vi "Vision Acquistion test.vi"() -> ()   [LabVIEW 2018]
uses:
  <vilib>/vision/driver/NI_Vision_Acquisition_Software.lvlib
panel:
  out "error out":errorcluster
  in  "error in":errorcluster
  in  "Stop (F)":bool
  out "Image Out":T1(plugin-control)
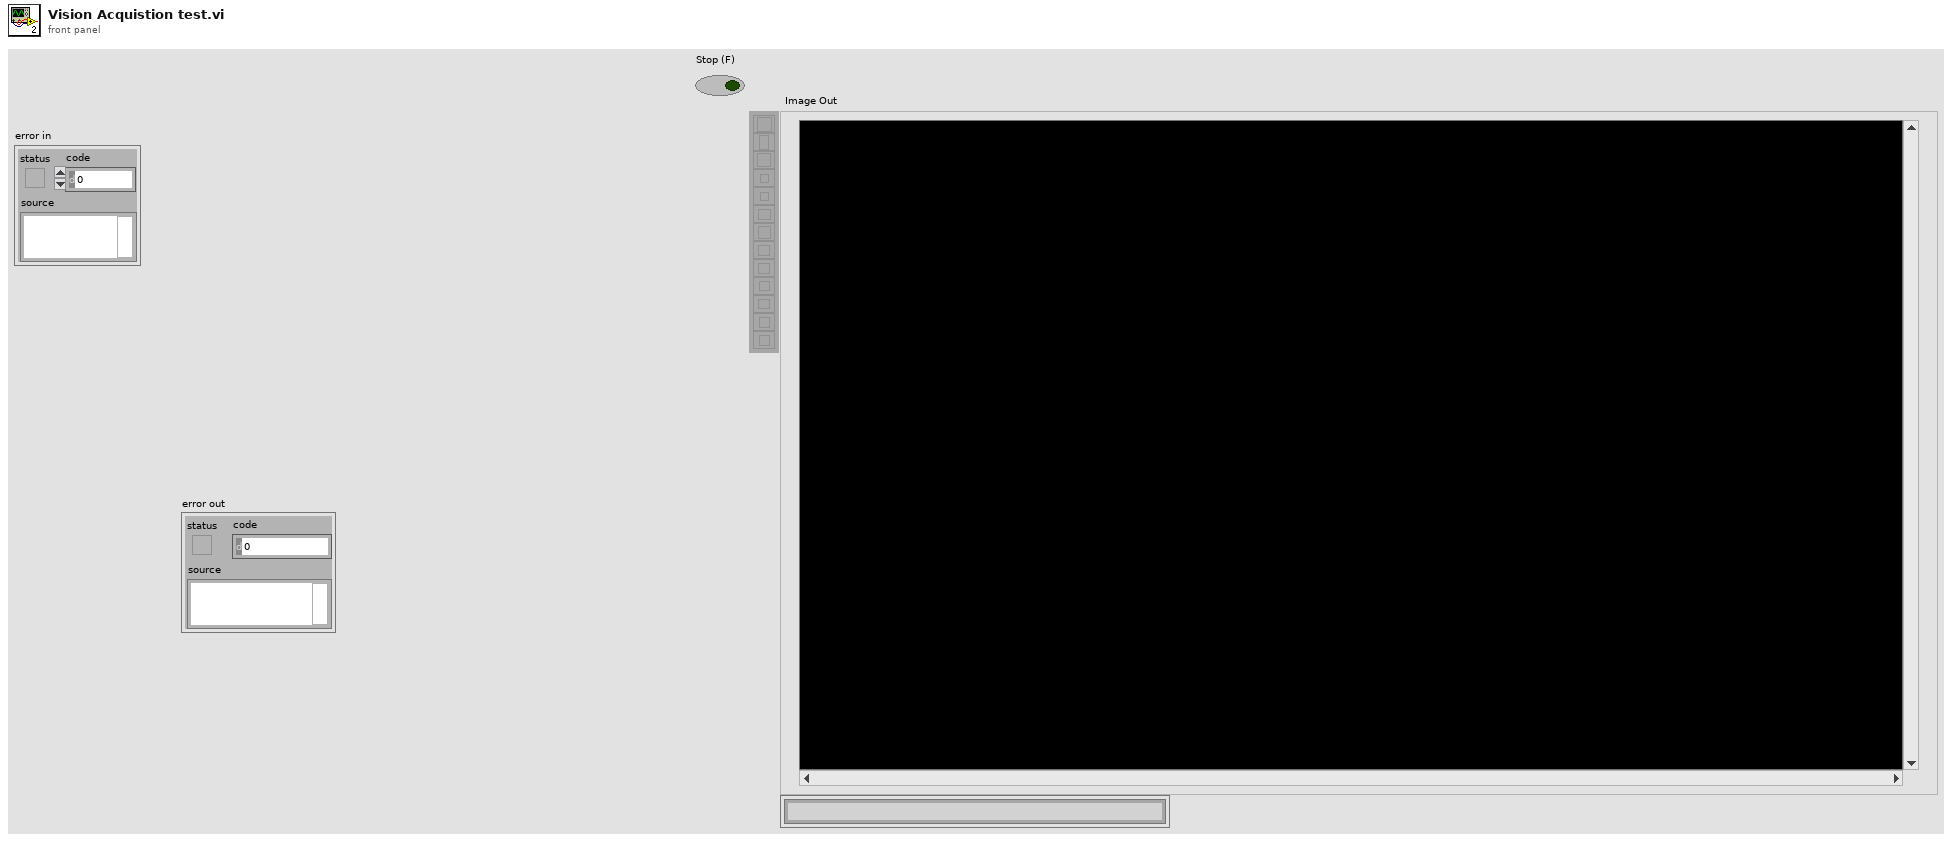
[diagram p1: front panel]
types:
  T1 = typedef "IMAQ Image.ctl" = refnum<image>
  T2 = typedef "IMAQdx.ctl" = refnum<k21>
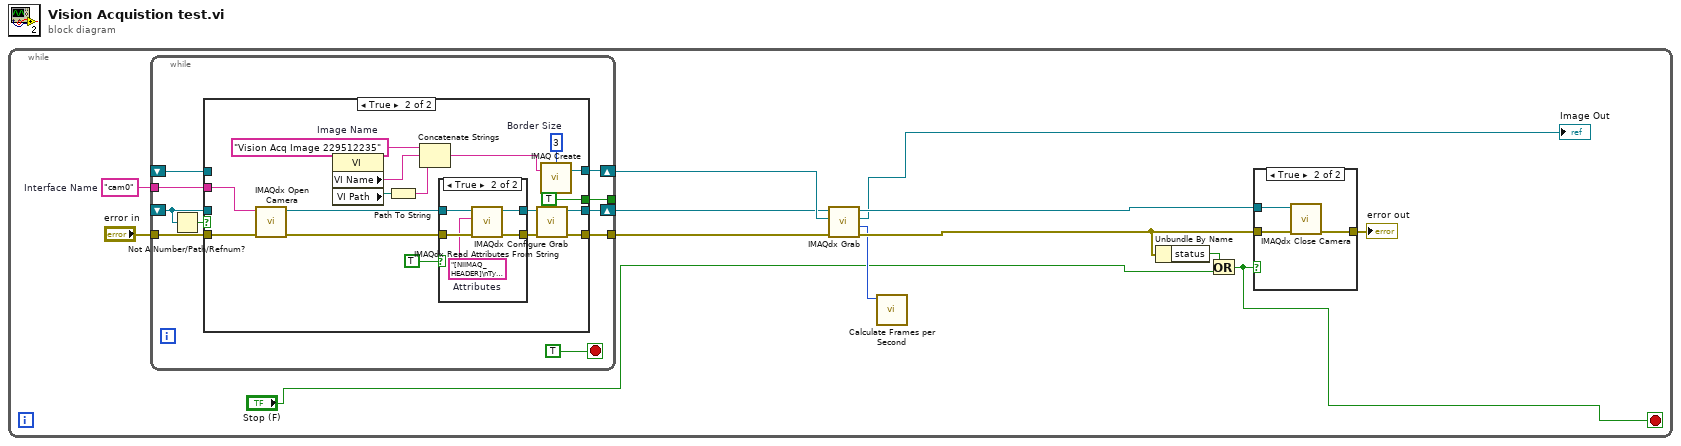
[diagram p0: block diagram]
diagram:
  n1 = while {
    stop <- w2 stop-if-true
    w11 = "cam0"  # Interface Name
    n2 = while "While Loop_template0" {
      shift-right: [w27] -> w9
      shift-left: _ -> [w20]
      tunnel: [w26] -> w12
      tunnel: "error in" -> [w25]
      shift-right: [w23] -> w10
      shift-left: _ -> [w22]
      tunnel: w11 -> [w21]
      tunnel: [w18] -> _
      stop <- TRUE ("_template0") stop-if-true
      n3 = Not A Number/Path/Refnum?(number/path/refnum=w20) -> (NaN/Path/Refnum?=w19:bool)
      n4 = case "Case Structure_template0" shown="True" w19 {
        tunnel: [w30 w46] -> w27
        tunnel: w20 -> [w30 _]
        tunnel: [w29 w45] -> w26
        tunnel: w25 -> [w29 w47]
        tunnel: [w28 w44] -> w23
        tunnel: w22 -> [w28 _]
        tunnel: w21 -> [_ w34]
        tunnel: [_ TRUE] -> w18
        frame False {
        }
        frame True {
          w31 = 3  # Border Size
          w39 = "Vision Acq Image 229512235"  # Image Name
          n5 = call <vilib>:"IMAQdx Open Camera.vi"("error in"=w47, "Session In"=w34) -> ("error out"=w37:errorcluster, "Session Out"=w38:T2)  [unwired: 1 in, 7 out]
          n6 = property class="VI"() -> ("VI Name"=w42:string, "VI Path"=w43:path)  [unwired: 2 in, 2 out]
          n7 = Path To String(path=w43) -> (string=w41:string)
          n8 = Concatenate Strings(w39, w42, w41) -> (w40:string)
          n9 = case shown="True" TRUE ("Init Attributes") {
            tunnel: w38 -> [w49 w54]
            tunnel: w37 -> [w48 w53]
            tunnel: [w49 w51] -> w36
            tunnel: [w48 w50] -> w35
            frame False {
            }
            frame True {
              w52 = "[NIIMAQ_HEADER]\nType = 2\nVersion = 8\n\n[CAMERA_DATA]\nAcquisitionAttributes::Bayer::Algorithm = \"Bilinear\"\nAcquisitionAttributes::Bayer::GainB = \"1\"\nAcquisitionAttributes::Bayer::GainG = \"1\"\nAcquisitionAttributes::Bayer::GainR = \"1\"\nAcquisitionAttributes::Bayer::Pattern = \"Use hardware value\"\nAcquisitionAttributes::BitsPerPixel = \"Use hardware value\"\nAcquisitionAttributes::HardwareMaximumQueuedBufferCount = \"1000\"\nAcquisitionAttributes::HardwareRequeueBufferListThreshold = \"50\"\nAcquisitionAttributes::IgnoreFirstFrame = \"false\"\nAcquisitionAttributes::ImageDecoderCopyMode = \"Auto\"\nAcquisitionAttributes::OutputImageType = \"Auto\"\nAcquisitionAttributes::OverwriteMode = \"Get Newest\"\nAcquisitionAttributes::PixelSignedness = \"Use hardware value\"\nAcquisitionAttributes::ReceiveTimestampMode = \"None\"\nAcquisitionAttributes::ShiftPixelBits = \"false\"\nAcquisitionAttributes::SwapPixelBytes = \"false\"\nAcquisitionAttributes::Timeout = \"5000\"\nAcquisitionAttributes::VideoMode = \"1920 x 1080 YUY 2 5.00 fps\"\nCameraAttributes::BacklightCompensation::Mode = \"Manual\"\nCameraAttributes::BacklightCompensation::Value = \"0\"\nCameraAttributes::Brightness::Mode = \"Manual\"\nCameraAttributes::Brightness::Value = \"168\"\nCameraAttributes::Contrast::Mode = \"Manual\"\nCameraAttributes::Contrast::Value = \"5\"\nCameraAttributes::Exposure::Mode = \"AutoAperaturePriority\"\nCameraAttributes::Focus::Mode = \"Auto\"\nCameraAttributes::Pan::Mode = \"Manual\"\nCameraAttributes::Pan::Value = \"0\"\nCameraAttributes::PowerLineFrequency::Mode = \"60Hz\"\nCameraAttributes::Saturation::Mode = \"Manual\"\nCameraAttributes::Saturation::Value = \"103\"\nCameraAttributes::Sharpness::Mode = \"Manual\"\nCameraAttributes::Sharpness::Value = \"25\"\nCameraAttributes::Tilt::Mode = \"Manual\"\nCameraAttributes::Tilt::Value = \"0\"\nCameraAttributes::WhiteBalance::Mode = \"Auto\"\nCameraAttributes::Zoom::Mode = \"Manual\"\nCameraAttributes::Zoom::Value = \"0\"\n"  # Attributes
              n10 = call <vilib>:"IMAQdx Read Attributes From String.vi"("error in"=w53, "Attributes String In"=w52, "Session In"=w54) -> ("error out"=w50:errorcluster, "Session Out"=w51:T2)  [unwired: 7 out]
            }
          }
          n11 = call <vilib>:"IMAQdx Configure Grab.vi"("error in"=w35, "Session In"=w36) -> ("error out"=w45:errorcluster, "Session Out"=w46:T2)  [unwired: 8 out]
          n12 = call "IMAQ Create"("Border Size"=w31, "Image Name"=w40) -> ("New Image"=w44:T1)  [unwired: 2 in, 2 out]
        }
      }
    }
    n13 = call <vilib>:"IMAQdx Grab.vi"("error in"=w12, "Image In"=w10, "Session In"=w9) -> ("error out"=w8:errorcluster, "Buffer Number Out"=w7:u32, "Image Out"=→"Image Out":T1, "Session Out"=w6:T2)  [unwired: 1 in, 4 out]
    n14 = call <vilib>:"Calculate Frames per Second.vi"("Buffer Number"=w7) -> ()  [unwired: 2 in, 9 out]
    n15 = Unbundle By Name(w8) -> ("status"=w4:bool)
    n16 = Or(x=w4, y="Stop (F)") -> (x .or. y?=w2:bool)
    n17 = case "Case Structure_template1" shown="True" w2 {
      tunnel: [w14 w16] -> w5
      tunnel: w8 -> [w14 w17]
      tunnel: w6 -> [_ w15]
      frame False {
      }
      frame True {
        n18 = call <vilib>:"IMAQdx Close Camera.vi"("error in"=w17, "Session In"=w15) -> ("error out"=w16:errorcluster)  [unwired: 9 out]
      }
    }
    "error out" <- w5
  }
